vi "TOML to LabVIEW.vi"(7 "Default Value":variant, 8 "error in (no error)":errorcluster, 10 "BlueSerializer in":refnum<class "BlueSerializer.lvclass">, 11 "TOML Value":T1) -> (0 "error out":errorcluster, 3 "LV Value":variant)   [LabVIEW 2019, in "BlueTOMLSerializer.lvlib"]
uses:
  BlueTOMLSerializer.lvlib
  TOML Value.ctl
  <userlib>/Blue Origin/BlueSerialization/BlueSerializer/BlueSerializer.lvclass
  Value.ctl
  Value Type.ctl
  Key-Value Pair.ctl
  Classes/BlueTOMLSerializer/StructuredData.ctl
  <vilib>/Utility/Data Type/NI_Data Type.lvlib
  Classes/BlueTOMLSerializer/BlueTOMLSerializer.lvclass
  <vilib>/JDP Science/JDP Science Common Utilities/JDP Utility.lvlib
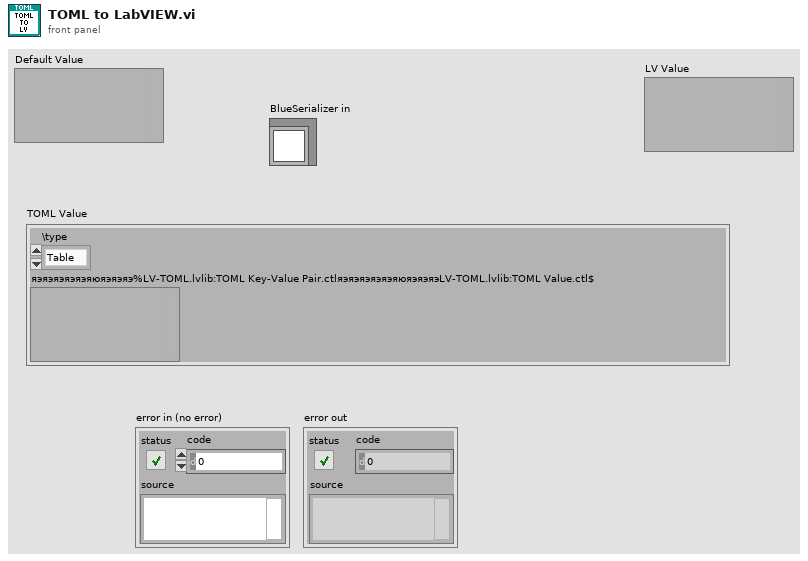
[diagram p1: front panel]
types:
  T1 = typedef "BlueTOMLSerializer.lvlib/TOML Value.ctl" = cluster{"\\type":enum16{"Table", "Array", "String", "Integer", "Float", "Boolean", "Offset Date-Time", "Local Date-Time", "Local Date", "Local Time"}, "яэяэяэяэяэяюяэяэяэ%LV-TOML.lvlib:TOML Key-Value Pair.ctlяэяэяэяэяэяюяэяэяэLV-TOML.lvlib:TOML Value.ctl$":variant}
  T2 = typedef "BlueTOMLSerializer.lvlib/Value.ctl" = cluster{"Type":T3, "Value":variant}
  T3 = typedef "BlueTOMLSerializer.lvlib/Value Type.ctl" = enum16{"Table", "Array", "String", "Integer", "Float", "Boolean", "Offset Date-Time", "Local Date-Time", "Local Date", "Local Time"}
  T4 = typedef "BlueTOMLSerializer.lvlib/Key-Value Pair.ctl" = cluster{"Key":string, "Value":T2}
  T5 = typedef "BlueTOMLSerializer.lvlib/BlueTOMLSerializer.lvclass/StructuredData.ctl" = cluster{"TOML Value":T1}
  T6 = typedef "NI_Data Type.lvlib/Data Type.ctl" = enum8{"Invalid Type", "Void", "I8", "I16", "I32", "I64", "U8", "U16", "U32", "U64", "Single Float", "Double Float", "Extended Float", "Single Complex", "Double Complex", "Extended Complex", "Enum U8", "Enum U16", "Enum U32", "Enum U64", "Single Float With Unit", "Double Float With Unit", "Extended Float With Unit", "Single Complex with Unit", "Double Complex with Unit", "Extended Complex with Unit", "Boolean", "String", "Path", "Picture", "Tag", "Array", "Cluster", "Variant", "LV Variant", "Waveform", "Timestamp", "Digital Waveform", "Digital Data", "ExpressData", "Refnum", "External Data", "VI", "Poly VI", "LabVIEW Class Instance", "Fixed Point", "Set Collection", "Map Collection"}
  T7 = typedef "NI_Data Type.lvlib/Memory Info.ctl" = cluster{"Type":T8, "Size":u32}
  T8 = typedef "NI_Data Type.lvlib/Memory Type.ctl" = enum16{"Variable", "Fixed", "Bounded"}
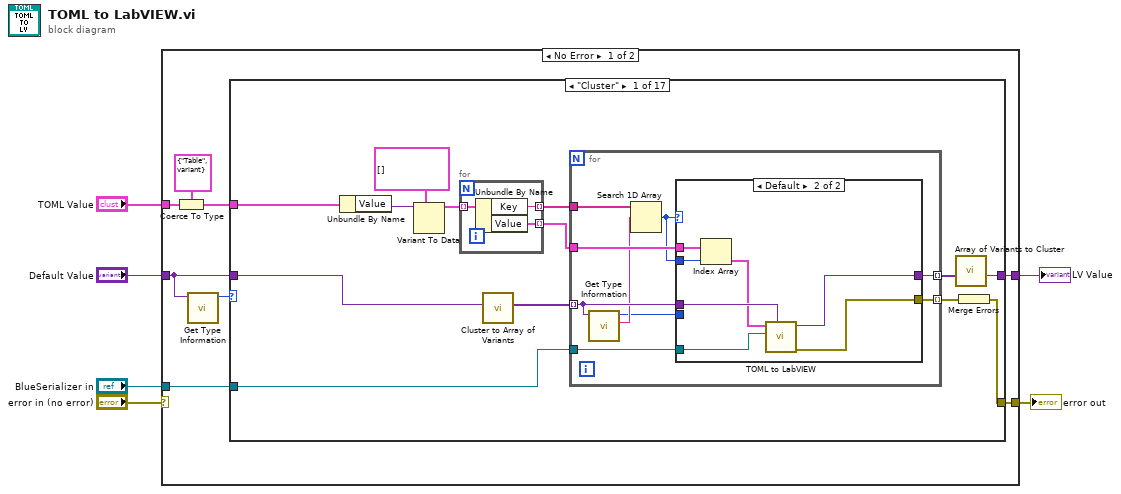
[diagram p0: block diagram]
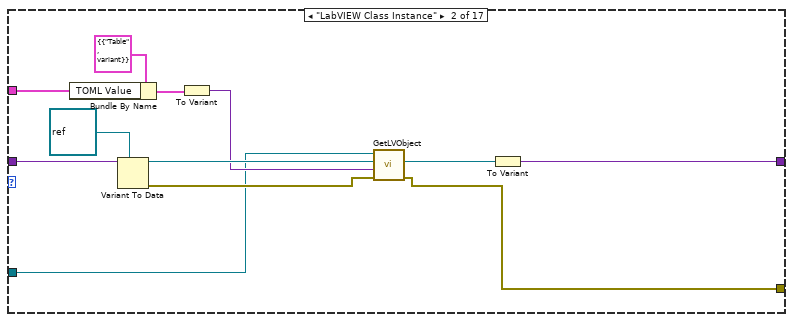
[diagram p3: hidden frame]
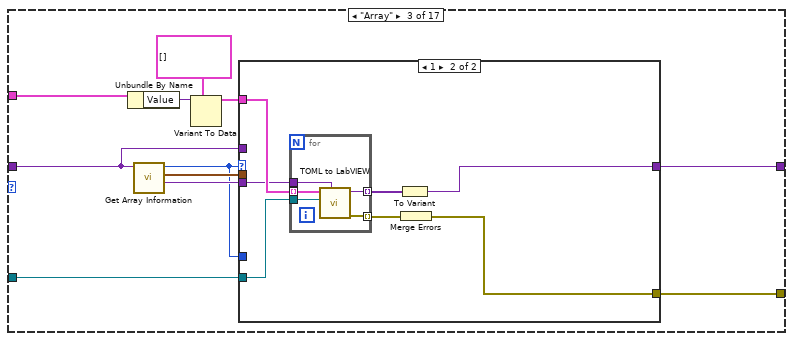
[diagram p4: hidden frame]
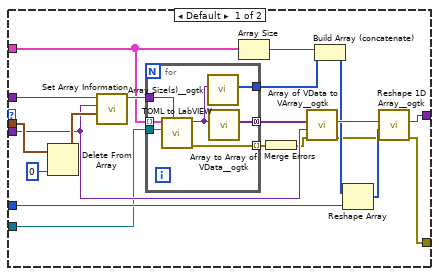
[diagram p5: hidden frame]
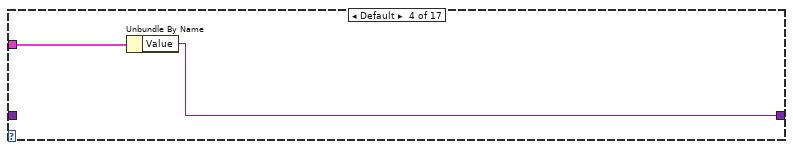
[diagram p6: hidden frame]
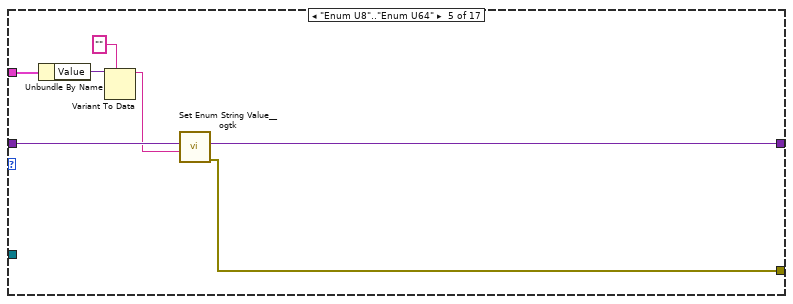
[diagram p7: hidden frame]
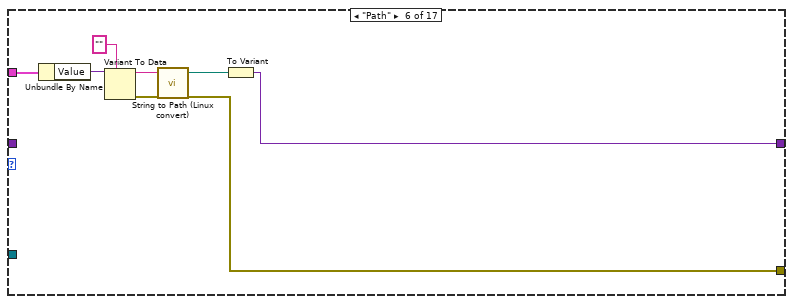
[diagram p8: hidden frame]
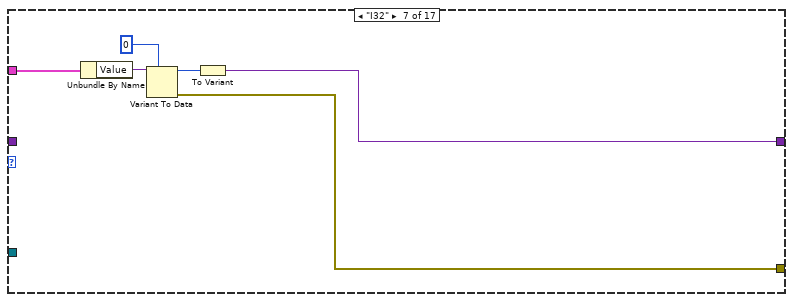
[diagram p9: hidden frame]
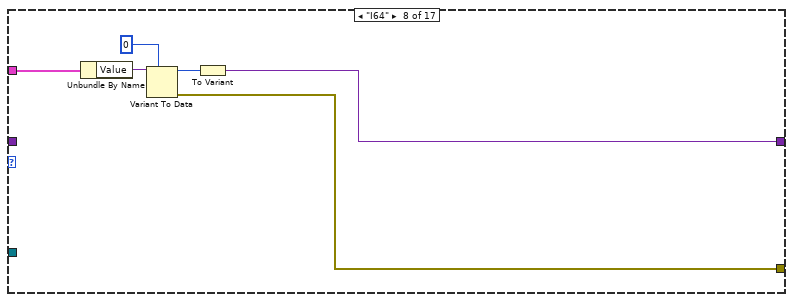
[diagram p10: hidden frame]
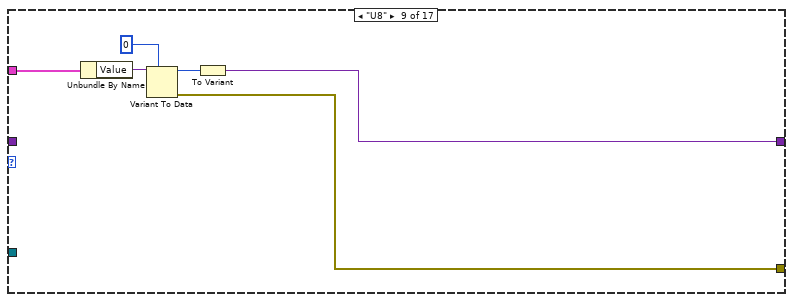
[diagram p11: hidden frame]
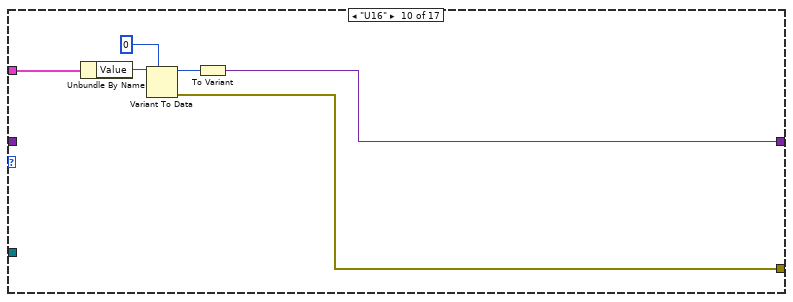
[diagram p12: hidden frame]
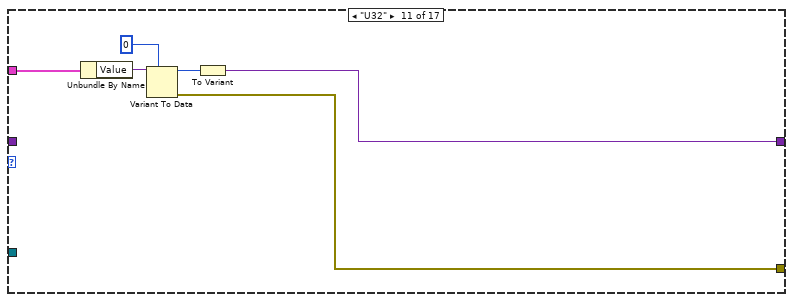
[diagram p13: hidden frame]
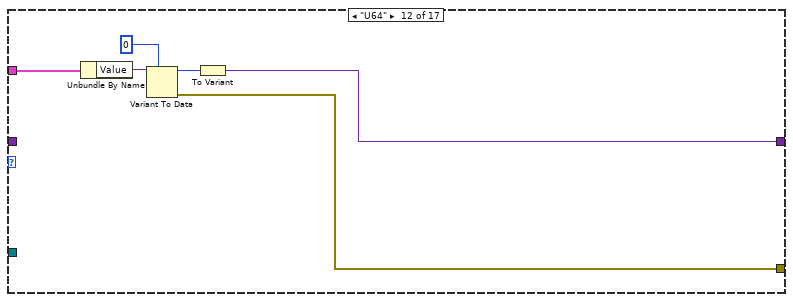
[diagram p14: hidden frame]
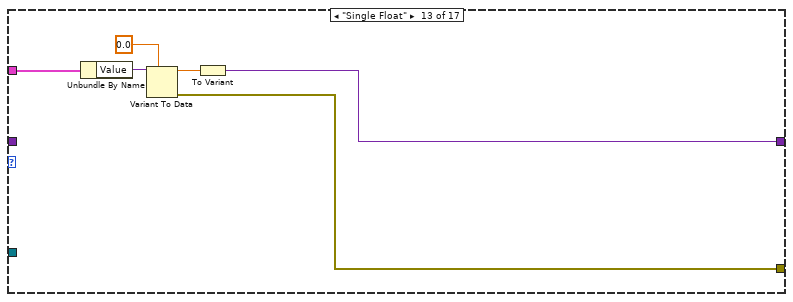
[diagram p15: hidden frame]
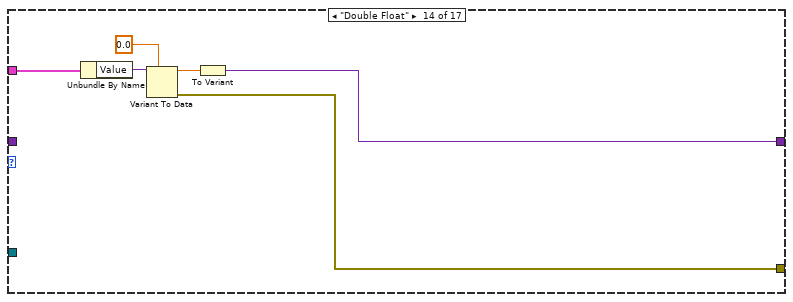
[diagram p16: hidden frame]
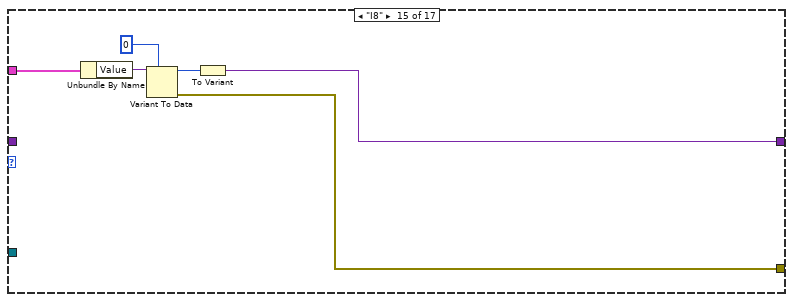
[diagram p17: hidden frame]
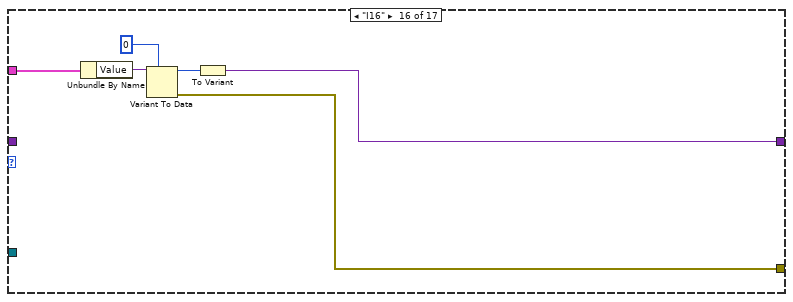
[diagram p18: hidden frame]
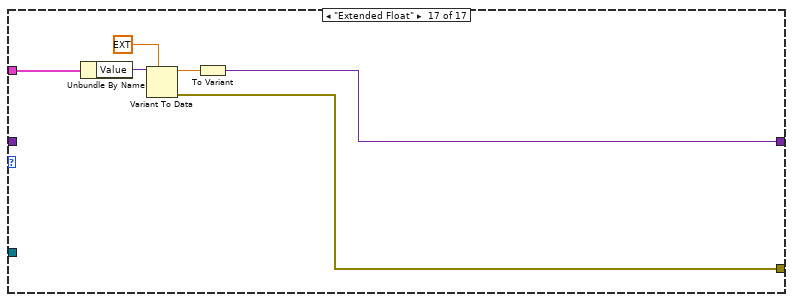
[diagram p19: hidden frame]
diagram:
  n1 = case shown="No Error" "error in (no error)" {
    selector: "error in (no error)" -> [_ w192]
    tunnel: "Default Value" -> [w13 _]
    tunnel: [w12 _] -> w5
    tunnel: "TOML Value" -> [w11 _]
    tunnel: [w8 w192] -> w2
    tunnel: "BlueSerializer in" -> [w7 _]
    frame No Error {
      n2 = Coerce To Type(0:w11, 1:T2 {"Type"=enum."Table", "Value"=variant} ("type")) -> (2:w10:T2)
      n3 = call <vilib>:"Get Type Information.vi"("variant"=w13) -> ("type"=w14:T6)  [unwired: 6 in, 4 out]
      n4 = case shown="\"Cluster\"" w14 {
        tunnel: w10 -> [w27 w50 w70 w111 w118 w125 w130 w136 w142 w148 w154 w160 w166 w172 w178 w184 w190]
        tunnel: w13 -> [w17 w59 w66 _ w115 _ _ _ _ _ _ _ _ _ _ _ _]
        tunnel: [w18 w54 w63 w110 w113 w122 w127 w133 w139 w145 w151 w157 w163 w169 w175 w181 w187] -> w12
        tunnel: [w20 w56 w61 _ w112 w121 w126 w132 w138 w144 w150 w156 w162 w168 w174 w180 w186] -> w8
        tunnel: w7 -> [w15 w48 w60 _ _ _ _ _ _ _ _ _ _ _ _ _ _]
        frame "Cluster" {
          n5 = Unbundle By Name(w27) -> ("Value"=w26:variant)
          n6 = Variant To Data(type=T4[] [], Variant=w26) -> (data=w23:T4[])  [unwired: 1 in, 1 out]
          n7 = for {
            tunnel: w23 -> [w30] mode=indexing
            tunnel: [w29] -> w24 mode=indexing
            tunnel: [w28] -> w22 mode=indexing
            n8 = Unbundle By Name(w30) -> ("Key"=w29:string, "Value"=w28:T2)
          }
          n9 = call <vilib>:"Cluster to Array of Variants.vi"("Cluster"=w17) -> ("Array of Cluster Elements"=w16:variant[])  [unwired: 10 in]
          n10 = for {
            tunnel: w16 -> [w37] mode=indexing
            tunnel: w24 -> [w39]
            tunnel: w22 -> [w38]
            tunnel: [w34] -> w21 mode=indexing
            tunnel: [w32] -> w19 mode=indexing
            tunnel: w15 -> [w31]
            n11 = call <vilib>:"Get Type Information.vi"("variant"=w37) -> ("name"=w36:string, "type"=w33:T6)  [unwired: 6 in, 3 out]
            n12 = Search 1D Array(1D array=w39, element=w36) -> (index of element=w35:i32)  [unwired: 1 in]
            n13 = case shown="Default" w35 {
              tunnel: w38 -> [_ w47]
              tunnel: w35 -> [_ w46]
              tunnel: [w40 w43] -> w32
              tunnel: w37 -> [w40 w45]
              tunnel: [_ w42] -> w34
              tunnel: w33 -> [_ _]
              tunnel: w31 -> [_ w41]
              frame -1 {
              }
              frame Default {
                n14 = Index Array(array=w47, index=w46) -> (element=w44:T2)
                n15 = call "TOML to LabVIEW.vi"("Default Value"=w45, "BlueSerializer in"=w41, "TOML Value"=w44) -> ("error out"=w42:errorcluster, "LV Value"=w43:variant)  [unwired: 7 in]
              }
            }
          }
          n16 = call <vilib>:"Array of Variants to Cluster.vi"("Array of Variants"=w19) -> ("Cluster of Variants"=w18:variant)  [unwired: 10 in]
          n17 = Merge Errors(w21) -> (w20:errorcluster)
        }
        frame "LabVIEW Class Instance" {
          n18 = Bundle By Name(cluster=T5 {"TOML Value"={"\\type"=enum."Table", "яэяэяэяэяэяюяэяэяэ%LV-TOML.lvlib:TOML Key-Value Pair.ctlяэяэяэяэяэяюяэяэяэLV-TOML.lvlib:TOML Value.ctl$"=variant}} ("Cluster"), "TOML Value"=w50) -> (w49:T5)
          n19 = Variant To Data(type=refnum<class> refnum ("LabVIEW Object"), Variant=w59) -> (data=w57:refnum<class>, error out=w52:errorcluster)  [unwired: 1 in]
          n20 = To Variant(anything=w49) -> (Variant=w53:variant)
          n21 = call <userlib>:"GetLVObject.vi"("error in (no error)"=w52, "StructuredData in"=w53, "Object Type"=w57, "BlueSerializer in"=w48) -> ("error out"=w56:errorcluster, "Object out"=w55:refnum<class>)  [unwired: 4 in, 2 out]
          n22 = To Variant(anything=w55) -> (Variant=w54:variant)
        }
        frame "Array" {
          n23 = Unbundle By Name(w70) -> ("Value"=w69:variant)
          n24 = call <vilib>:"Get Array Information.vi"("variant"=w66) -> ("array element data type"=w67:variant, "array lengths"=w65:T7[], "number of dimensions"=w62:i32)  [unwired: 7 in, 1 out]
          n25 = Variant To Data(type=T2[] [], Variant=w69) -> (data=w64:T2[])  [unwired: 1 in, 1 out]
          n26 = case shown="1" w62 {
            tunnel: w67 -> [w79 w103]
            tunnel: w66 -> [w90 _]
            tunnel: w65 -> [w89 _]
            tunnel: w64 -> [w85 w104]
            tunnel: [w82 w100] -> w63
            tunnel: w62 -> [w78 _]
            tunnel: [w72 w99] -> w61
            tunnel: w60 -> [w71 w98]
            frame Default {
              n27 = Delete From Array(array=w89, index=0) -> (array with subset deleted=w87:T7[])  [unwired: 1 in, 1 out]
              n28 = call <vilib>:"Set Array Information.vi"("Array Lengths"=w87, "Array Element"=w79, "Variant in"=w90) -> ("Variant out"=w86:variant)  [unwired: 7 in, 1 out]
              n29 = for {
                tunnel: w86 -> [w97]
                tunnel: w85 -> [w94] mode=indexing
                tunnel: [w96] -> w83
                tunnel: [w95] -> w81 mode=concatenating
                tunnel: [w92] -> w75 mode=indexing
                tunnel: w71 -> [w91]
                n30 = call "TOML to LabVIEW.vi"("Default Value"=w97, "BlueSerializer in"=w91, "TOML Value"=w94) -> ("error out"=w92:errorcluster, "LV Value"=w93:variant)  [unwired: 7 in]
                n31 = call <userlib>:"Array Size(s)__ogtk.vi"("Array"=w93) -> ("Size(s)"=w96:u32[])  [unwired: 8 in, 2 out]
                n32 = call <userlib>:"Array to Array of VData__ogtk.vi"("MultiD Array"=w93) -> ("1D Array of Variants"=w95:variant[])  [unwired: 9 in, 1 out]
              }
              n33 = Array Size(array=w85) -> (size(s)=w84:i32)
              n34 = Merge Errors(w75) -> (w74:errorcluster)
              n35 = call <userlib>:"Array of VData to VArray__ogtk.vi"("error in (no error)"=w74, "Element Type (when empty)"=w79, "1D Array of VData"=w81) -> ("error out"=w73:errorcluster, "VArray"=w80:variant)  [unwired: 7 in]
              n36 = Build Array (concatenate)(w84, w83) -> (w77:u32[])
              n37 = Reshape Array(w77, w78) -> (w76:u32[])
              n38 = call <userlib>:"Reshape 1D Array__ogtk.vi"("error in (no error)"=w73, "Size(s)"=w76, "1D Array"=w80) -> ("error out"=w72:errorcluster, "Reshaped VArray"=w82:variant)  [unwired: 7 in]
            }
            frame 1 {
              n39 = for {
                tunnel: w103 -> [w109]
                tunnel: w104 -> [w108] mode=indexing
                tunnel: [w107] -> w101 mode=indexing
                tunnel: [w106] -> w102 mode=indexing
                tunnel: w98 -> [w105]
                n40 = call "TOML to LabVIEW.vi"("Default Value"=w109, "BlueSerializer in"=w105, "TOML Value"=w108) -> ("error out"=w106:errorcluster, "LV Value"=w107:variant)  [unwired: 7 in]
              }
              n41 = To Variant(anything=w101) -> (Variant=w100:variant)
              n42 = Merge Errors(w102) -> (w99:errorcluster)
            }
          }
        }
        frame Default {
          n43 = Unbundle By Name(w111) -> ("Value"=w110:variant)
        }
        frame "Enum U8".."Enum U64" {
          n44 = Unbundle By Name(w118) -> ("Value"=w117:variant)
          n45 = Variant To Data(type="", Variant=w117) -> (data=w114:string)  [unwired: 1 in, 1 out]
          n46 = call <userlib>:"Set Enum String Value__ogtk.vi"("String Value"=w114, "Default Enum Value"=w115) -> ("error out"=w112:errorcluster, "Enum"=w113:variant)  [unwired: 8 in]
        }
        frame "Path" {
          n47 = Unbundle By Name(w125) -> ("Value"=w124:variant)
          n48 = Variant To Data(type="", Variant=w124) -> (data=w120:string, error out=w121:errorcluster)  [unwired: 1 in]
          n49 = call "String to Path (Linux convert).vi"("Windows path"=w120) -> ("Path"=w119:path)  [unwired: 4 in]
          n50 = To Variant(anything=w119) -> (Variant=w122:variant)
        }
        frame "I32" {
          n51 = Unbundle By Name(w130) -> ("Value"=w131:variant)
          n52 = Variant To Data(type=0, Variant=w131) -> (data=w128:i32, error out=w126:errorcluster)  [unwired: 1 in]
          n53 = To Variant(anything=w128) -> (Variant=w127:variant)
        }
        frame "I64" {
          n54 = Unbundle By Name(w136) -> ("Value"=w137:variant)
          n55 = Variant To Data(type=i64 0, Variant=w137) -> (data=w134:i64, error out=w132:errorcluster)  [unwired: 1 in]
          n56 = To Variant(anything=w134) -> (Variant=w133:variant)
        }
        frame "U8" {
          n57 = Unbundle By Name(w142) -> ("Value"=w143:variant)
          n58 = Variant To Data(type=u8 0, Variant=w143) -> (data=w140:u8, error out=w138:errorcluster)  [unwired: 1 in]
          n59 = To Variant(anything=w140) -> (Variant=w139:variant)
        }
        frame "U16" {
          n60 = Unbundle By Name(w148) -> ("Value"=w149:variant)
          n61 = Variant To Data(type=u16 0, Variant=w149) -> (data=w146:u16, error out=w144:errorcluster)  [unwired: 1 in]
          n62 = To Variant(anything=w146) -> (Variant=w145:variant)
        }
        frame "U32" {
          n63 = Unbundle By Name(w154) -> ("Value"=w155:variant)
          n64 = Variant To Data(type=u32 0, Variant=w155) -> (data=w152:u32, error out=w150:errorcluster)  [unwired: 1 in]
          n65 = To Variant(anything=w152) -> (Variant=w151:variant)
        }
        frame "U64" {
          n66 = Unbundle By Name(w160) -> ("Value"=w161:variant)
          n67 = Variant To Data(type=u64 0, Variant=w161) -> (data=w158:u64, error out=w156:errorcluster)  [unwired: 1 in]
          n68 = To Variant(anything=w158) -> (Variant=w157:variant)
        }
        frame "Single Float" {
          n69 = Unbundle By Name(w166) -> ("Value"=w167:variant)
          n70 = Variant To Data(type=sgl 0.0, Variant=w167) -> (data=w164:sgl, error out=w162:errorcluster)  [unwired: 1 in]
          n71 = To Variant(anything=w164) -> (Variant=w163:variant)
        }
        frame "Double Float" {
          n72 = Unbundle By Name(w172) -> ("Value"=w173:variant)
          n73 = Variant To Data(type=0.0, Variant=w173) -> (data=w170:dbl, error out=w168:errorcluster)  [unwired: 1 in]
          n74 = To Variant(anything=w170) -> (Variant=w169:variant)
        }
        frame "I8" {
          n75 = Unbundle By Name(w178) -> ("Value"=w179:variant)
          n76 = Variant To Data(type=i8 0, Variant=w179) -> (data=w176:i8, error out=w174:errorcluster)  [unwired: 1 in]
          n77 = To Variant(anything=w176) -> (Variant=w175:variant)
        }
        frame "I16" {
          n78 = Unbundle By Name(w184) -> ("Value"=w185:variant)
          n79 = Variant To Data(type=i16 0, Variant=w185) -> (data=w182:i16, error out=w180:errorcluster)  [unwired: 1 in]
          n80 = To Variant(anything=w182) -> (Variant=w181:variant)
        }
        frame "Extended Float" {
          n81 = Unbundle By Name(w190) -> ("Value"=w191:variant)
          n82 = Variant To Data(type=ext 0.0, Variant=w191) -> (data=w188:ext, error out=w186:errorcluster)  [unwired: 1 in]
          n83 = To Variant(anything=w188) -> (Variant=w187:variant)
        }
      }
    }
    frame Error {
    }
  }
  "LV Value" <- w5
  "error out" <- w2
